vi "Command Turn to Target.vi"(2 "All Robot Commands In":T1, 3 "Startup":bool, 4 "Cmd Parameter 4":string, 5 "Cmd Parameter 3":dbl, 6 "Cmd Parameter 2":dbl, 7 "Cmd Parameter 1":dbl) -> (0 "All Robot Commands Out":T1, 1 "Completed":bool)   [LabVIEW 2016]
uses:
  Subsystems/All Robot Commands.ctl
  Subsystems/Drive and Climb SS/Drive + Climb Commands 2017.ctl
  Subsystems/Gear Delivery SS/Gear Delivery Commands.ctl
  Subsystems/Conveyor and Shooter SS/Conveyor and Shooter Commands.ctl
  Subsystems/Ball Intake SS/Ball Intake Commands.ctl
  Command Execution State.ctl
  Global Variables/Sensor Data.vi
  Robot Global Data.vi
panel:
  out "Calculated Target Heading":dbl
  out "Robot Heading":dbl
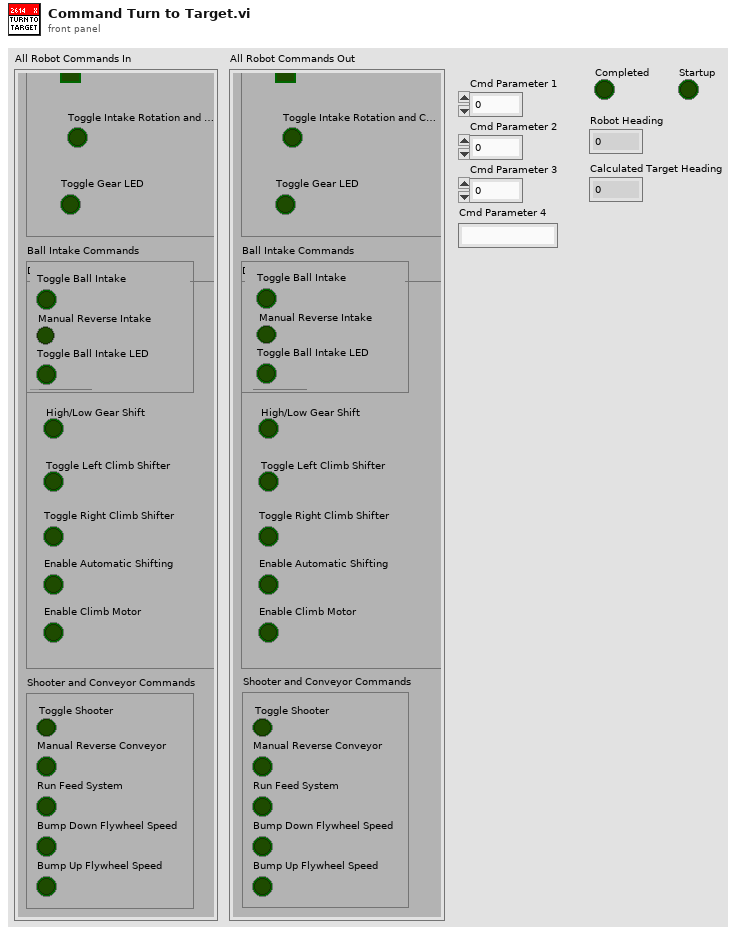
[diagram p1: front panel]
types:
  T1 = typedef "All Robot Commands.ctl" = cluster{"Drive/Climb Commands":T2, "Gear Delivery Commands":T3, "Shooter and Conveyor Commands":T4, "Ball Intake Commands":T5}
  T2 = typedef "Drive + Climb Commands 2017.ctl" = cluster{"Robot Forward-Back":dbl, "Robot Twist":dbl, "High/Low Gear Shift":bool, "Toggle Left Climb Shifter":bool, "Toggle Right Climb Shifter":bool, "Enable Automatic Shifting":bool, "Enable Climb Motor ":bool}
  T3 = typedef "Gear Delivery Commands.ctl" = cluster{"Toggle Gear Release":bool, "Toggle Intake Rotation and Chute Door":bool, "Toggle Gear LED":bool}
  T4 = typedef "Conveyor and Shooter Commands.ctl" = cluster{"Toggle Shooter":bool, "Manual Reverse Conveyor":bool, "Run Feed System":bool, "Bump Down Flywheel Speed":bool, "Bump Up Flywheel Speed":bool}
  T5 = typedef "Ball Intake Commands.ctl" = cluster{"Toggle Ball Intake":bool, "Manual Reverse Intake":bool, "Toggle Ball Intake LED":bool}
  T6 = typedef "Command Execution State.ctl" = enum16{"Initialize", "Execute", "Finish"}
  T7 = cluster{"Distance (ft)":dbl, "Score":dbl, "Normalized":cluster{"Center":cluster{dbl, dbl}, "Rectangle":cluster{"Numeric":dbl, "Numeric 2":dbl, "Numeric 3":dbl, "Numeric 5":dbl}}, "Pixels":cluster{"Center":cluster{dbl, dbl}, "Rectangle":cluster{"Numeric":dbl, "Numeric 2":dbl, "Numeric 3":dbl, "Numeric 5":dbl}}}
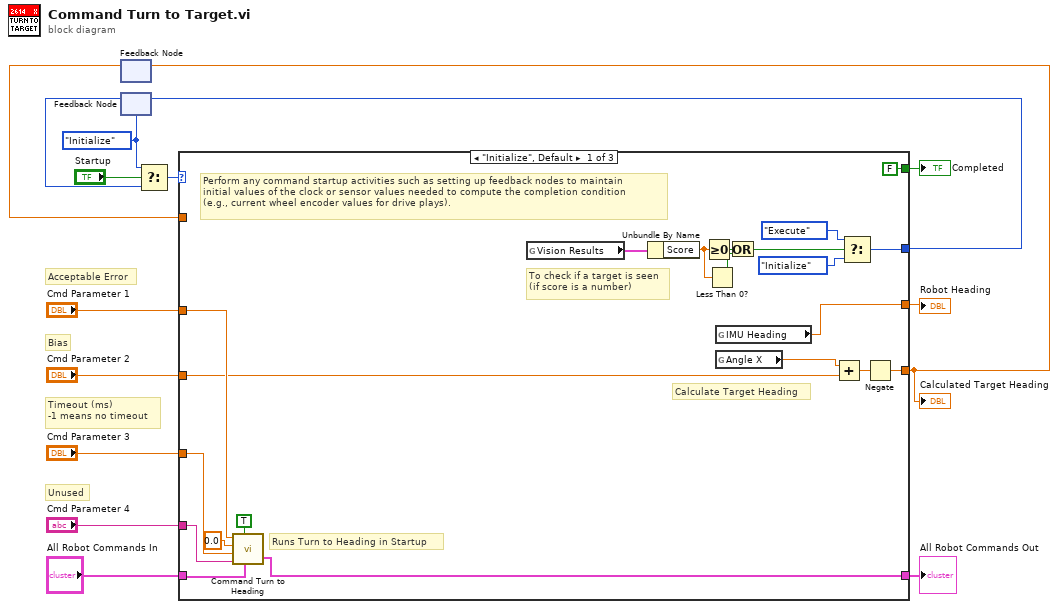
[diagram p0: block diagram]
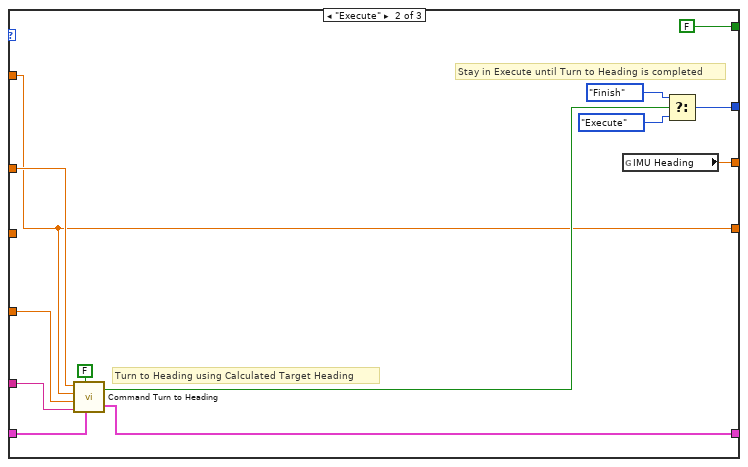
[diagram p2: hidden frame]
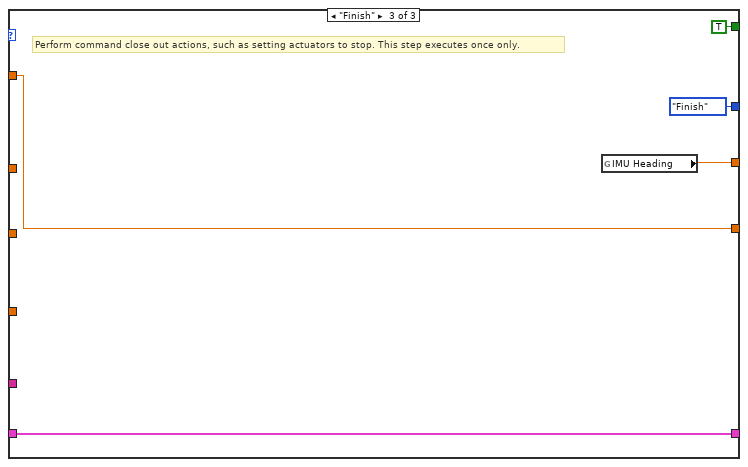
[diagram p3: hidden frame]
diagram:
  w7 = Command_Execution_State."Initialize" ("Play State")
  # "Unused"
  # "Timeout (ms)\n-1 means no timeout"
  # "Bias"
  # "Acceptable Error"
  n1 = feedback #1() -> (w2:dbl)  [unwired: 1 in]
  n2 = feedback #2(w7) -> (w9:T6)
  n3 = Select(t=w7, s="Startup", f=w9) -> (s? t:f=w8:T6)
  n4 = case shown="\"Initialize\", Default" w8 {
    tunnel: [FALSE FALSE TRUE] -> w15
    tunnel: [w30 w48 Command_Execution_State."Finish" ("f")] -> w14
    tunnel: "Cmd Parameter 1" -> [w29 w44 _]
    tunnel: "Cmd Parameter 2" -> [w25 _ _]
    tunnel: "Cmd Parameter 3" -> [w28 w43 _]
    tunnel: "Cmd Parameter 4" -> [w27 w42 _]
    tunnel: [w22 w45 w53] -> w3
    tunnel: [w24 w41 w52] -> w5
    tunnel: "All Robot Commands In" -> [w35 w38 w52]
    tunnel: w2 -> [_ w37 w51]
    tunnel: [w17 w37 w51] -> w1
    frame "Initialize", Default {
      # "To check if a target is seen\n(if score is a number)"
      # "Runs Turn to Heading in Startup"
      # "Calculate Target Heading"
      # "Perform any command startup activities such as setting up feedback nodes to maintain \ninitial values of the clock or sensor values needed to compute the completion condition\n(e.g., current wheel encoder values for drive plays)."
      n5 = call "Command Turn to Heading.vi"("All Robot Commands In"=w35, "Startup"=TRUE, "Cmd Parameter 4"=w27, "Cmd Parameter 3"=w28, "Cmd Parameter 2"=0.0, "Cmd Parameter 1"=w29) -> ("All Robot Commands Out"=w24:T1)  [unwired: 1 out]
      n6 = global read "Robot Global Data.vi" "Vision Results"() -> (w23:T7)
      n7 = Unbundle By Name(w23) -> ("Score"=w18:dbl)
      n8 = Greater Or Equal To 0?(x=w18) -> (x >= 0?=w20:bool)
      n9 = Less Than 0?(x=w18) -> (x < 0?=w19:bool)
      n10 = global read "Sensor Data.vi" "IMU Heading"() -> (w22:dbl)
      n11 = global read "Sensor Data.vi" "Angle X"() -> (w16:dbl)
      n12 = Or(x=w20, y=w19) -> (x .or. y?=w21:bool)
      n13 = Add(x=w16, y=w25) -> (x+y=w26:dbl)
      n14 = Select(t=Command_Execution_State."Execute" ("Play State"), s=w21, f=Command_Execution_State."Initialize" ("Play State")) -> (s? t:f=w30:T6)
      n15 = Negate(x=w26) -> (-x=w17:dbl)
    }
    frame "Execute" {
      # "Stay in Execute until Turn to Heading is completed"
      # "Turn to Heading using Calculated Target Heading"
      n16 = call "Command Turn to Heading.vi"("All Robot Commands In"=w38, "Startup"=FALSE, "Cmd Parameter 4"=w42, "Cmd Parameter 3"=w43, "Cmd Parameter 2"=w37, "Cmd Parameter 1"=w44) -> ("All Robot Commands Out"=w41:T1, "Completed"=w40:bool)
      n17 = global read "Sensor Data.vi" "IMU Heading"() -> (w45:dbl)
      n18 = Select(t=Command_Execution_State."Finish" ("Play State"), s=w40, f=Command_Execution_State."Execute" ("Play State")) -> (s? t:f=w48:T6)
    }
    frame "Finish" {
      # "Perform command close out actions, such as setting actuators to stop. This step executes once only."
      n19 = global read "Sensor Data.vi" "IMU Heading"() -> (w53:dbl)
    }
  }
  "Completed" <- w15
  "Robot Heading" <- w3
  "All Robot Commands Out" <- w5
  "Calculated Target Heading" <- w1
  n20 = feedback-in #1(w1) -> ()
  n21 = feedback-in #2(w14) -> ()
